vi "SpeedFilter (1).vi"(2 "error in (no error)":errorcluster, 3 "Raw Signal":dbl) -> (0 "error out":errorcluster, 1 "Filtered Signal":dbl)   [LabVIEW 2013]
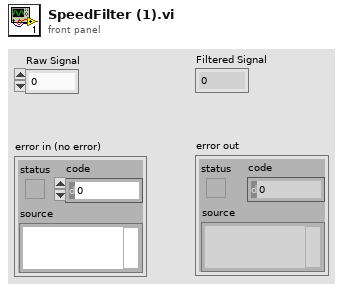
[diagram p1: front panel]
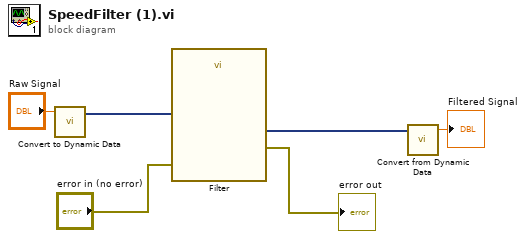
[diagram p0: block diagram]
diagram:
  n1 = call "Convert to Dynamic Data"("Double"="Raw Signal") -> ("Dynamic Data Type"=w6:dynamicdata)  [unwired: 3 in]
  n2 = call "Filter"("error in (no error)"="error in (no error)", "Signal"=w6) -> ("error out"=→"error out":errorcluster, "Filtered Signal"=w3:dynamicdata)  [unwired: 8 in]
  n3 = call "Convert from Dynamic Data"("Dynamic Data Type"=w3) -> ("Scalar"=→"Filtered Signal":dbl)  [unwired: 3 in]
